vi "Get DDG Insertion Delay.vi"(8 "error in (no error)":errorcluster, 11 "piState":i32) -> (0 "error out":errorcluster, 2 "function return":u32, 3 "piState out":i32)   [LabVIEW 2014, in "atmcd32d.lvlib"]
doc: "unsigned int WINAPI GetDDGInsertionDelay(int * piState);"
uses:
  atmcd32d.lvlib
  atmcd32d.dll
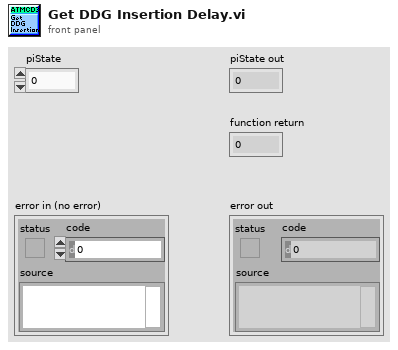
[diagram p1: front panel]
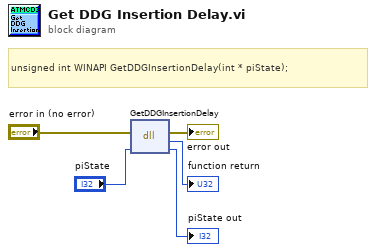
[diagram p0: block diagram]
diagram:
  # "unsigned int WINAPI GetDDGInsertionDelay(int * piState);"
  n1 = dll-call lib="C:/Users/Bakir/Documents/Lambda2-Testing/lib/Andorlib/atmcd32d.*" fn="GetDDGInsertionDelay"(error in="error in (no error)", "piState"="piState") -> (error out=→"error out":errorcluster, →"function return":u32, "piState"=→"piState out":i32)  [unwired: 2 in, 1 out]
